vi "Pfeiffer Vacuum Turbo Operating adjustment.vi"(8 "error in (no error)":errorcluster, 10 "Adress of unit":u16=1 min=1 max=999 step=1, 11 "COM Port Name in":refnum<visa-resource-name>="COM1") -> (0 "error out":errorcluster, 3 "response (data)":string)   [LabVIEW 2016]
doc: "This VI is an example of how to use the Pfeiffer Vacuum subVIs programmatically. This VI first initializes the instrument, takes measurements, then closes the instrument."
uses:
  Public/Turbopumps/PV Operating adjustment - Cluster.ctl
  Pfeiffer Vacuum.lvlib
panel:
  in  "Operating adjustment - Cluster":T1={"Parameter"=0, "Parameter\nread only<->describe"=FALSE, "off<->on"=TRUE, "Rotation speed set value\nin rot. speed setting\noperations [%]"=50.0, "Preset rotation Speed\nat Standby mode (%)"=66.0, "maximum power\nsetpoint [%]"=100, "Gas mode"=0} {"Gas mode" items=["heavy gases", "light gases", "helium"]; "maximum power\nsetpoint [%]" min=10 max=100 step=1; "Preset rotation Speed\nat Standby mode (%)" min=20.0 max=100.0 step=0.1 format="%.2f"; "Rotation speed set value\nin rot. speed setting\noperations [%]" min=20.0 max=100.0 step=0.1 format="%.2f"; "Parameter" items=[" Standby", " Pumping station", " Motor Turbopump", " Oper. mode TMP", " Gas mode", " Operating mode drive unit", " Rotation speed set value in rot. speed setting operations", " Set rotation speed TMP [Hz] (read only)", " Actual rotation speed TMP [Hz] (read only)", " Preset rotation Speed at Standby mode (%)", " Max. rotations speed ", " maximum power setpoint"]}
  # "Standby                                     :\n Pumping station                      :     \n Motor turbopump                    :\n Operations mode TMP           :\n Operating mode drive unit   :"
  # "<--------------\n  off\n  off\n  off\n  final rot. speed oper.       \n  max."
  # "----------->                 \non \non \non \nrot. speed setting \n reduced power consumpt."
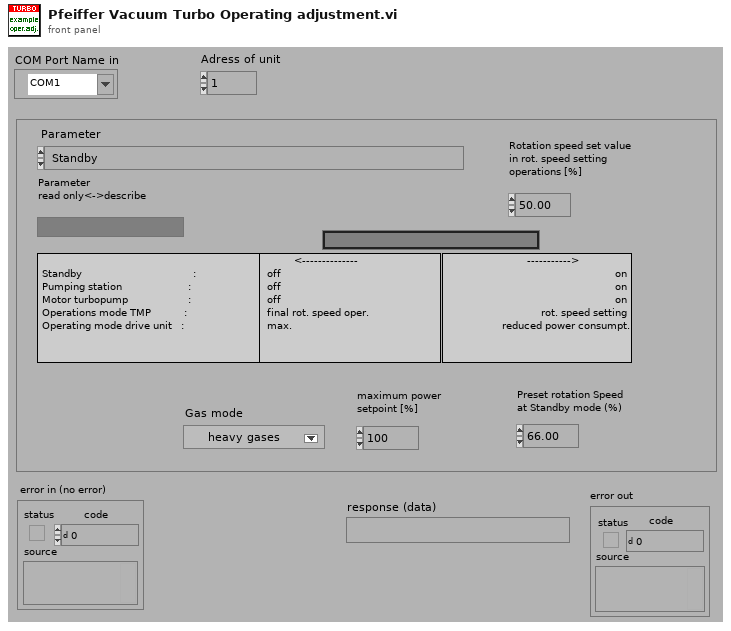
[diagram p1: front panel]
types:
  T1 = typedef "Pfeiffer Vacuum.lvlib/PV Operating adjustment - Cluster.ctl" = cluster{"Parameter":u16, "Parameter\nread only<->describe":bool, "off<->on":bool, "Rotation speed set value\nin rot. speed setting\noperations [%]":dbl, "Preset rotation Speed\nat Standby mode (%)":dbl, "maximum power\nsetpoint [%]":i32, "Gas mode":u16}
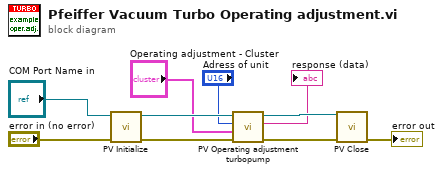
[diagram p0: block diagram]
diagram:
  n1 = call "PV Initialize.vi"("error in (no error)"="error in (no error)", "VISA session in"="COM Port Name in") -> ("error out"=w10:errorcluster, "VISA session out"=w8:refnum<visa-resource-name>)  [unwired: 8 in]
  n2 = call "PV Operating adjustment turbopump.vi"("error in (no error)"=w10, "Operating adjustment - Cluster"="Operating adjustment - Cluster", "Adress of unit"="Adress of unit", "VISA session"=w8) -> ("error out"=w9:errorcluster, "response (data)"=→"response (data)":string, "dup VISA session"=w7:refnum<visa-resource-name>)  [unwired: 5 in]
  n3 = call "PV Close.vi"("VISA session"=w7, "error in (no error)"=w9) -> ("error out"=→"error out":errorcluster)  [unwired: 13 in]
